vi "ErrorCheckHWI.vi"(8 "error in (no error)":errorcluster, 11 "Slave_Line in":refnum<class "Slave_Line.lvclass">) -> (0 "error out":errorcluster, 3 "Slave_Line out":refnum<class "Slave_Line.lvclass">)   [LabVIEW 2013, in "Slave_Line.lvclass"]
uses:
  Slave_Line.lvclass
  Device/Device.lvclass
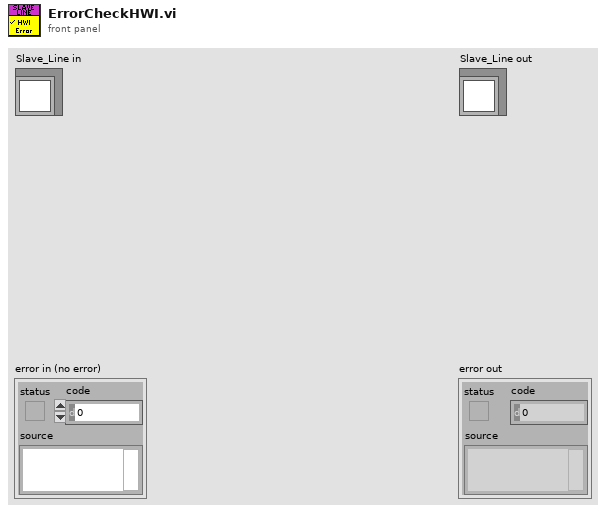
[diagram p1: front panel]
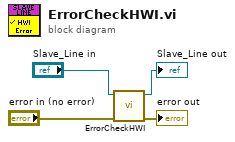
[diagram p0: block diagram]
diagram:
  n1 = call-parent "ErrorCheckHWI.vi"("error in (no error)"="error in (no error)", "Device in"="Slave_Line in") -> ("error out"=→"error out":errorcluster, "Device out"=→"Slave_Line out":refnum<class "Slave_Line.lvclass">)  [unwired: 8 in]
